vi "WS1021_FPGA MEMS Only Initialize.vi"(8 "Error In":errorcluster, 10 "FPGA":T4, 11 "Active Log":refnum<vi>) -> (0 "Error Out":errorcluster, 3 "System Out":T1={"Settings"={"I2C Slave Address"=144, "I2C Clock Rate (Hz)"=20.0, "SRL Clock Rate (Hz)"=50000.0, "Simulate FPGA"=TRUE, "C1 Cap DAC Default"=165, "C2 Cap DAC Default"=165, "C3 Cap DAC Default"=134, "C4 Cap DAC Default"=150, "DAC Out Vref (V)"=0.0}, "FPGA Resource"="", "Online"=FALSE, "I2C Wait Ticks"=0, "SRL Wait Ticks"=0, "FPGA VI Reference (FPGA Mode)"=refnum, "FPGA VI Reference (Sim Mode)"=refnum} {"Settings"."DAC Out Vref (V)" format="%.3f V"; "Settings"."C4 Cap DAC Default" format="0x%02x"; "Settings"."C3 Cap DAC Default" format="0x%02x"; "Settings"."C2 Cap DAC Default" format="0x%02x"; "Settings"."C1 Cap DAC Default" format="0x%02x"; "Settings"."SRL Clock Rate (Hz)" format="%.0f Hz"; "Settings"."I2C Clock Rate (Hz)" format="%.0f Hz"; "Settings"."I2C Slave Address" format="0x%02x"})   [LabVIEW 2017]
uses:
  WS_VCAP Driver 1_49/Source/WSVCAP Shell/Type Defs/WSVCAP SHL FPGA Enum.ctl
  WS_VCAP Driver 1_49/Source/WSVCAP Shell/Type Defs/WSVCAP SHL Core System Cluster.ctl
  WS_VCAP Driver 1_49/Source/WSVCAP Shell/Type Defs/WSVCAP SHL I2C Settings Cluster.ctl
  WS_VCAP Driver 1_49/Source/WSVCAP Shell/Type Defs/WSVCAP SHL FPGA Ref.ctl
  WS_VCAP Driver 1_49/Source/WSVCAP Shell/Type Defs/Cap and DAC Table Manager Operation Enum.ctl
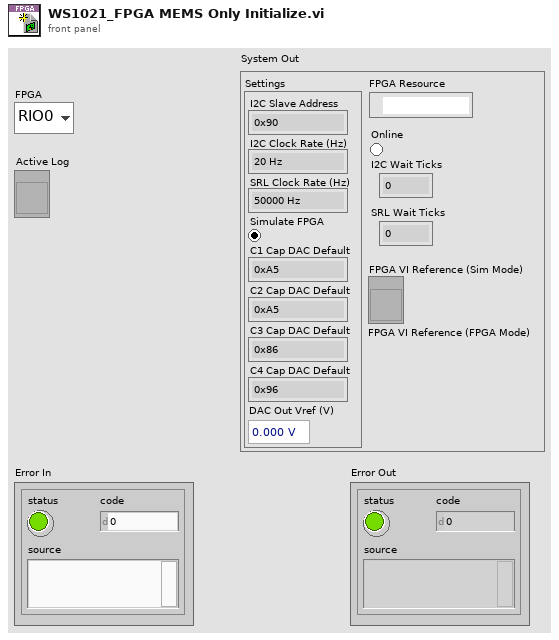
[diagram p1: front panel]
types:
  T1 = typedef "WSVCAP SHL Core System Cluster.ctl" = cluster{"Settings":T2, "FPGA Resource":tag, "Online":bool, "I2C Wait Ticks":u32, "SRL Wait Ticks":u32, "FPGA VI Reference (FPGA Mode)":T3, "FPGA VI Reference (Sim Mode)":refnum<vi>}
  T2 = typedef "WSVCAP SHL I2C Settings Cluster.ctl" = cluster{"I2C Slave Address":u8, "I2C Clock Rate (Hz)":dbl, "SRL Clock Rate (Hz)":dbl, "Simulate FPGA":bool, "C1 Cap DAC Default":u8, "C2 Cap DAC Default":u8, "C3 Cap DAC Default":u8, "C4 Cap DAC Default":u8, "DAC Out Vref (V)":dbl}
  T3 = typedef "WSVCAP SHL FPGA Ref.ctl" = refnum<k20>
  T4 = typedef "WSVCAP SHL FPGA Enum.ctl" = enum16{"RIO0", "RIO1"}
  T5 = typedef "Cap and DAC Table Manager Operation Enum.ctl" = enum16{"Initialize", "Add Single DAC", "Add All DAC", "Add All DUT Single DAC", "Add All Cap", "Get Status"}
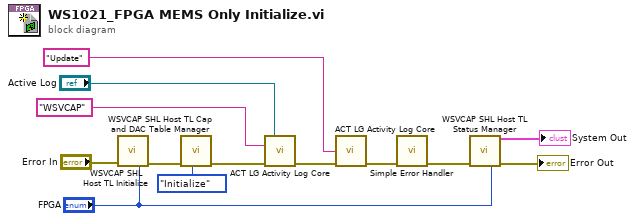
[diagram p0: block diagram]
diagram:
  n1 = call "WSVCAP SHL Host TL Initialize.vi"("error in"="Error In", "FPGA"="FPGA") -> ("error out"=w12:errorcluster)  [unwired: 12 in, 1 out]
  n2 = call "WSVCAP SHL Host TL Cap and DAC Table Manager.vi"("Operation"=Cap_and_DAC_Table_Manager_Operation_Enum."Initialize", "Error In"=w12) -> ("Error Out"=w7:errorcluster)  [unwired: 8 in, 1 out]
  n3 = call "ACT LG Activity Log Core.vi"("Display Ref"="Active Log", "Source"="WSVCAP", "Error In (no error)"=w7) -> ("Error Out"=w6:errorcluster)  [unwired: 11 in, 1 out]
  n4 = call "ACT LG Activity Log Core.vi"("Log Line"="Update", "Error In (no error)"=w6) -> ("Error Out"=w4:errorcluster)  [unwired: 12 in, 1 out]
  n5 = call <vilib>:"Simple Error Handler.vi"("error in (no error)"=w4) -> ("error out"=w5:errorcluster)  [unwired: 4 in, 4 out]
  n6 = call "WSVCAP SHL Host TL Status Manager.vi"("error in"=w5, "FPGA"="FPGA") -> ("System Out"=→"System Out":T1, "error out"=→"Error Out":errorcluster)  [unwired: 12 in]
